vi "Load Plugin Management Core.vi"(11 "CIFPluginManager in":refnum<class "CIFPluginManager.lvclass">) -> (0 "error out":errorcluster)   [LabVIEW 2021, in "CIFPluginManager.lvclass"]
uses:
  CIFPluginManager.lvclass
  CIFPluginManager.lvclass/CIFPluginManager.ctl
  gRPC/CIF_Manager_server/RPC Service/Manager/Manager.lvclass
  C:/Program Files/National Instruments/LabVIEW 2021/vi.lib/gRPC/LabVIEW gRPC Servicer/ServiceBase/ServiceBase.lvclass
  gRPC/CIF_Manager_server/RPC Service/Manager/Manager.lvclass/Manager.ctl
  gRPC/CIF_Manager_server/RPC Messages/cif_manager_LoadPluginResponse.ctl
  gRPC/CIF_Manager_server/RPC Messages/cif_common_Status.ctl
  typedef/Plugin Load Command.ctl
  typedef/Loader Type.ctl
  <vilib>/Utility/miscctls.llb/LVMapReplaceAction.ctl
  <vilib>/CIF Foundation/CIF Core/CIFCore/Common/Typedef/Errors.ctl
  typedef/Loader Load Command.ctl
  gRPC/CIF_Manager_server/RPC Messages/cif_manager_AbortPluginResponse.ctl
  gRPC/CIF_Manager_server/RPC Messages/cif_manager_AbortAllPluginsResponse.ctl
  gRPC/CIF_Manager_server/RPC Messages/Get cif_manager_LoadPluginRequest.vi
  gRPC/CIF_Manager_server/RPC Messages/Set cif_manager_LoadPluginResponse.vi
  <vilib>/CIF Foundation/CIF Utilities/Errors/Append Error Location.vi
  gRPC/CIF_Manager_server/RPC Messages/Get cif_manager_AbortPluginRequest.vi
  gRPC/CIF_Manager_server/RPC Messages/Set cif_manager_AbortPluginResponse.vi
  gRPC/CIF_Manager_server/RPC Messages/Get cif_manager_AbortAllPluginsRequest.vi
  gRPC/CIF_Manager_server/RPC Messages/Set cif_manager_AbortAllPluginsResponse.vi
  gRPC/CIF_Manager_server/RPC Messages/Get cif_manager_LoadPluginRequest.vi/2ed25e12-861d-4677-8ead-ace2906b2041.vi
  gRPC/CIF_Manager_server/RPC Messages/FlatToRichcif_manager_LoadPluginRequest.vi
  gRPC/CIF_Manager_server/RPC Messages/Set cif_manager_LoadPluginResponse.vi/dcc74a39-081a-4bdd-860b-8ed792803c96.vi
  gRPC/CIF_Manager_server/RPC Messages/RichToFlatcif_manager_LoadPluginResponse.vi
  gRPC/CIF_Manager_server/RPC Messages/Get cif_manager_AbortPluginRequest.vi/2ed25e12-861d-4677-8ead-ace2906b2041.vi
  gRPC/CIF_Manager_server/RPC Messages/FlatToRichcif_manager_AbortPluginRequest.vi
  gRPC/CIF_Manager_server/RPC Messages/Set cif_manager_AbortPluginResponse.vi/dcc74a39-081a-4bdd-860b-8ed792803c96.vi
  gRPC/CIF_Manager_server/RPC Messages/RichToFlatcif_manager_AbortPluginResponse.vi
  gRPC/CIF_Manager_server/RPC Messages/Get cif_manager_AbortAllPluginsRequest.vi/2ed25e12-861d-4677-8ead-ace2906b2041.vi
  gRPC/CIF_Manager_server/RPC Messages/FlatToRichcif_manager_AbortAllPluginsRequest.vi
  gRPC/CIF_Manager_server/RPC Messages/Set cif_manager_AbortAllPluginsResponse.vi/dcc74a39-081a-4bdd-860b-8ed792803c96.vi
  gRPC/CIF_Manager_server/RPC Messages/RichToFlatcif_manager_AbortAllPluginsResponse.vi
  <vilib>/gRPC/LabVIEW gRPC Library/Shared/TranslateGrpcError.vi
  gRPC/CIF_Manager_server/RPC Messages/RichToFlatcif_common_Status.vi
  <vilib>/gRPC/LabVIEW gRPC Library/Server API/Server/Get Server DLL Path.vi
  <vilib>/Utility/error.llb/Error Cluster From Error Code.vi
  <vilib>/string/Create NI GUID.vi
  <vilib>/gRPC/LabVIEW gRPC Library/Server API/Message Requests/Complete Call.vi
  <vilib>/CIF Foundation/CIF Core/CIFUtilities/CIFLogs/CIFLogs.lvlib
  <vilib>/CIF Foundation/CIF Core/CIFCore/Common/CIFCoreCommon.lvlib
  <vilib>/CIF Foundation/CIF Core/CIFCore/Grpc/CIFCoreWrapper/CIFCoreWrapper.lvlib
  <vilib>/CIF Foundation/CIF Utilities/Time/Time_CIF_U.lvlib
  <vilib>/CIF Foundation/CIF Core/CIFPluginManager/gRPC/CIF_Manager_Client_Wrapper/CIFManagerClientWrapper.lvlib
  CIFPluginLoader/gRPC/CIF_Plugin_Loader_Client_Wrapper/CIFPluginLoaderClientWrapper.lvlib
  gRPC/CIF_Manager_server/CIF_Manager_server.lvlib
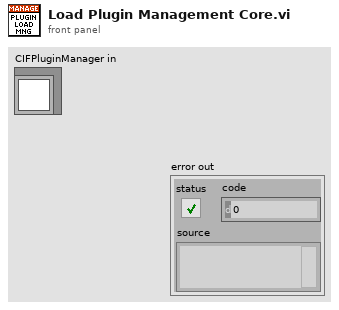
[diagram p1: front panel]
types:
  T1 = typedef "CIF_Manager_server.lvlib/Manager.lvclass/Server gRPC UEs.ctl" = cluster{"Manager LoadPlugin gRPC UE":refnum<user-event>, "Manager RegisterPlugin gRPC UE":refnum<user-event>, "Manager UnregisterPlugin gRPC UE":refnum<user-event>, "Manager QueryPluginTypes gRPC UE":refnum<user-event>, "Manager AbortPlugin gRPC UE":refnum<user-event>, "Manager UnloadAllPlugins gRPC UE":refnum<user-event>, "Manager Destroy gRPC UE":refnum<user-event>, "Manager Ping gRPC UE":refnum<user-event>, "Manager QueryErrors gRPC UE":refnum<user-event>, "Manager QueryConfig gRPC UE":refnum<user-event>, "Manager QueryInfo gRPC UE":refnum<user-event>, "Manager ResetErrorIndex gRPC UE":refnum<user-event>, "Manager ResetConfigIndex gRPC UE":refnum<user-event>, "Manager ResetInfoIndex gRPC UE":refnum<user-event>, "Manager QueryPluginInfo gRPC UE":refnum<user-event>, "Manager QueryPlugin gRPC UE":refnum<user-event>, "Manager QuerySystemStatus gRPC UE":refnum<user-event>, "Manager UpdateClock gRPC UE":refnum<user-event>, "Manager CreateOrch gRPC UE":refnum<user-event>, "Manager QueryClockStatus gRPC UE":refnum<user-event>, "Manager QueryAllChannels gRPC UE":refnum<user-event>, "Manager RegisterPluginLoader gRPC UE":refnum<user-event>, "Manager UnregisterPluginLoader gRPC UE":refnum<user-event>, "Manager CreatePluginLoader gRPC UE":refnum<user-event>, "Manager DestroyPluginLoader gRPC UE":refnum<user-event>, "Manager QueryPluginLoaders gRPC UE":refnum<user-event>}
  T2 = typedef "CIF_Manager_server.lvlib/cif_manager_LoadPluginResponse.ctl" = cluster{"status":T3}
  T3 = typedef "CIF_Manager_server.lvlib/cif_common_Status.ctl" = cluster{"code":i32, "message":string}
  T4 = typedef "CIFPluginManager.lvclass/Plugin Load Command.ctl" = cluster{"Plugin Name":string, "Plugin Path":string, "Loader Name":string, "Loader Type":T5}
  T5 = typedef "CIFPluginManager.lvclass/Loader Type.ctl" = enum16{"LabVIEW"}
  T6 = typedef "LVMapReplaceAction.ctl" = enum32{"Modify Entry only if found", "Add or Modify Entry", "Delete Entry"}
  T7 = typedef "CIFCoreCommon.lvlib/Errors.ctl" = enum16{"Invalid Clock ID", "Long Sleep", "gRPC Server Not Found", "Config Parse", "Timestamp Wrap", "Delayed Execution", "Duplicate Channel", "Missing Channel", "Incorrect Type", "Flatten Error", "Unflatten Data", "Unique Name", "Plugin Not Found", "Plugin Type Not Found", "Plugin Version Not Found", "Manager Not Found", "Numerical Issue", "Time Jump", "Clock ID Match", "Channel Length", "Plugin Connection", "gRPC Server Connection", "PPL Name Match", "Build", "Config Log Parse", "Plugin Load", "UI Subpanel Load", "Python Name", "Invalid Name", "Unable to Change Ch Buffer", "Failed Kill", "Failed SysExec", "Function Not Implemented", "Load Timeout"}
  T8 = typedef "CIFPluginManager.lvclass/Loader Load Command.ctl" = cluster{"Loader Type":T5, "Loader Name":string}
  T9 = typedef "CIF_Manager_server.lvlib/cif_manager_AbortPluginResponse.ctl" = cluster{"status":T3}
  T10 = typedef "CIF_Manager_server.lvlib/cif_manager_AbortAllPluginsResponse.ctl" = cluster{"status":T3}
  T11 = typedef "grpc-lvsupport-release.lvlib/grpcId.ctl" = u64
  T12 = typedef "CIF_Manager_server.lvlib/cif_manager_LoadPluginRequest.ctl" = cluster{"plugin_type":string, "plugin_name":string, "version":string, "loader_process":string}
  T13 = typedef "CIFPluginManager.lvclass/Discovered Plugin.ctl" = cluster{"Filename":string, "Plugin Type":string, "Qualified name":string, "Version":T14, "Plugin Metadata":T15, "Loader Type":T5, "File Path":string, "Relative Path":string[]}
  T14 = typedef "CIFCoreCommon.lvlib/Version.ctl" = cluster{"Major":i32, "Minor":i32, "Fix":i32, "Build":i32}
  T15 = typedef "CIFPluginManager.lvclass/Plugin Metadata.ctl" = cluster{"Description":string, "History":string, "Author":string}
  T16 = typedef "CIF_Manager_client.lvlib/cif_common_Status.ctl" = cluster{"code":i32, "message":string}
  T17 = typedef "CIFPluginManager.lvclass/Loader Map.ctl" = map{string, T18}
  T18 = typedef "CIFPluginManager.lvclass/Loaders.ctl" = cluster{"Loader Type":T5, "grpc_port":i32, "pid":u32, "gRPC ID":T11, "Load Timestamp":i64, "Unloading":bool, "Ready for removal":bool, "Unload Timestamp":i64}
  T19 = typedef "CIFPluginManager.lvclass/Plugin Management Data Map.ctl" = map{string, T20}
  T20 = typedef "CIFPluginManager.lvclass/Plugin Management Data.ctl" = cluster{"Unique Name":string, "Plugin Type":string, "gRPC Port":i32, "gRPC ID":T11, "Loader Type":T5, "Loader":string, "Version":T14, "Load Timestamp":i64, "Unload Timestamp":i64, "Unloading":bool, "Ready for removal":bool, "status":T21, "channels":T30}
  T21 = typedef "CIF_Manager_server.lvlib/cif_management_common_PluginStatusData.ctl" = cluster{"state":T22, "timing_statistics":T23, "fifo_statistics":T25, "error":T26, "monitor_doubles":T27, "monitor_u64s":T28, "monitor_i64s":T29}
  T22 = typedef "CIF_Manager_server.lvlib/cif_management_common_PluginStatusData_PluginState.ctl" = enum32{"PLUGINSTATE_UNKNOWN", "PLUGINSTATE_CREATING", "PLUGINSTATE_LISTENING", "PLUGINSTATE_RUNNING", "PLUGINSTATE_CLEANINGUP", "PLUGINSTATE_DESTROYING"}
  T23 = typedef "CIF_Manager_server.lvlib/cif_management_common_TimingStatistics.ctl" = cluster{"period":T24, "wake_error":T24, "execute":T24, "housekeep":T24, "idle":T24, "cleanup":T24, "custom_1":T24, "custom_2":T24}
  T24 = typedef "CIF_Manager_server.lvlib/cif_common_TimingStats.ctl" = cluster{"max":i64, "min":i64, "avg":dbl}
  T25 = typedef "CIF_Manager_server.lvlib/cif_management_common_FifoStatistics.ctl" = cluster{"from_t0":T24, "from_previous_plugin":T24, "output_error":T24}
  T26 = typedef "CIF_Manager_server.lvlib/cif_management_common_Error.ctl" = cluster{"status":bool, "code":i32}
  T27 = typedef "CIF_Manager_server.lvlib/cif_management_common_MonitorDoubles.ctl" = cluster{"double_1":dbl, "double_2":dbl, "double_3":dbl, "double_4":dbl}
  T28 = typedef "CIF_Manager_server.lvlib/cif_management_common_MonitorU64.ctl" = cluster{"u64_1":u64, "u64_2":u64, "u64_3":u64, "u64_4":u64}
  T29 = typedef "CIF_Manager_server.lvlib/cif_management_common_MonitorI64.ctl" = cluster{"i64_1":i64, "i64_2":i64, "i64_3":i64, "i64_4":i64}
  T30 = typedef "CIF_Manager_server.lvlib/cif_management_common_Channels.ctl" = cluster{"channels":T31[]}
  T31 = typedef "CIF_Manager_server.lvlib/cif_management_common_Channel.ctl" = cluster{"name":string, "direction":T32, "type":string, "custom_config":u8[], "connected":bool, "connected_name":string, "forced":bool, "channel_pattern":T33}
  T32 = typedef "CIF_Manager_server.lvlib/cif_management_common_ChannelDirection.ctl" = enum32{"CHANNELDIRECTION_UNKNOWN", "CHANNELDIRECTION_PUBLISHER", "CHANNELDIRECTION_SUBSCRIBER"}
  T33 = typedef "CIF_Manager_server.lvlib/cif_management_common_ChannelPattern.ctl" = enum32{"CHANNELPATTERN_UNKNOWN", "CHANNELPATTERN_TAG", "CHANNELPATTERN_FIFO", "CHANNELPATTERN_MULTIFIFO", "CHANNELPATTERN_BACKPRESSUREFIFO"}
  T34 = typedef "CIF_Manager_server.lvlib/cif_manager_AbortPluginRequest.ctl" = cluster{"plugin_name":string}
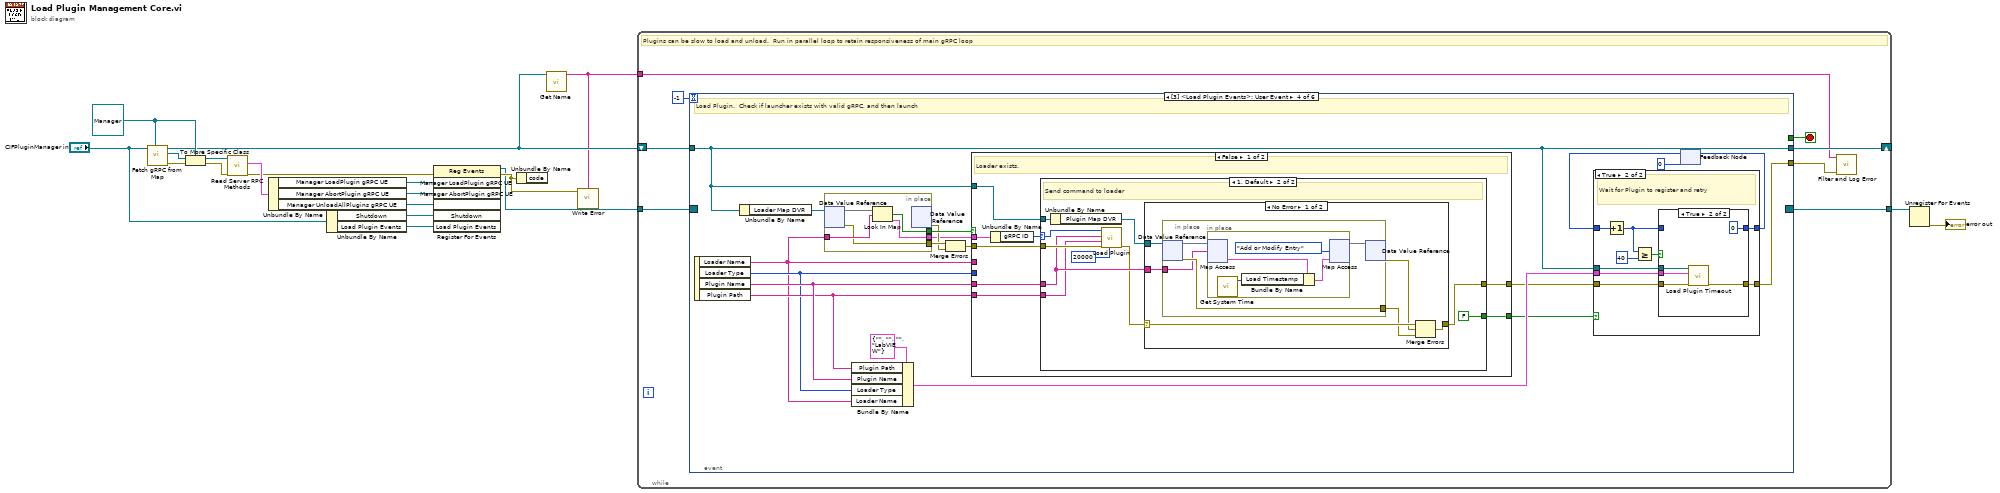
[diagram p0: block diagram]
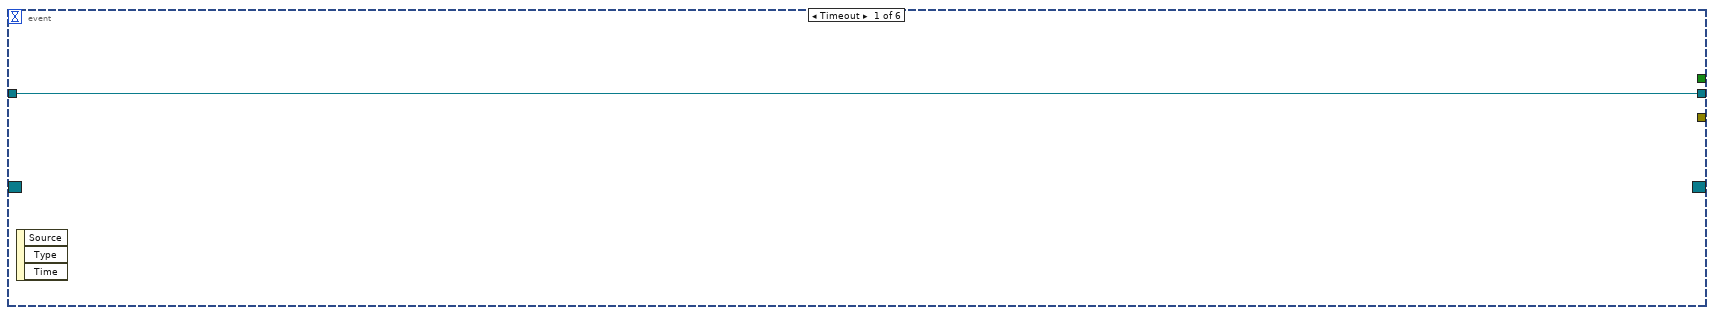
[diagram p2: hidden frame]
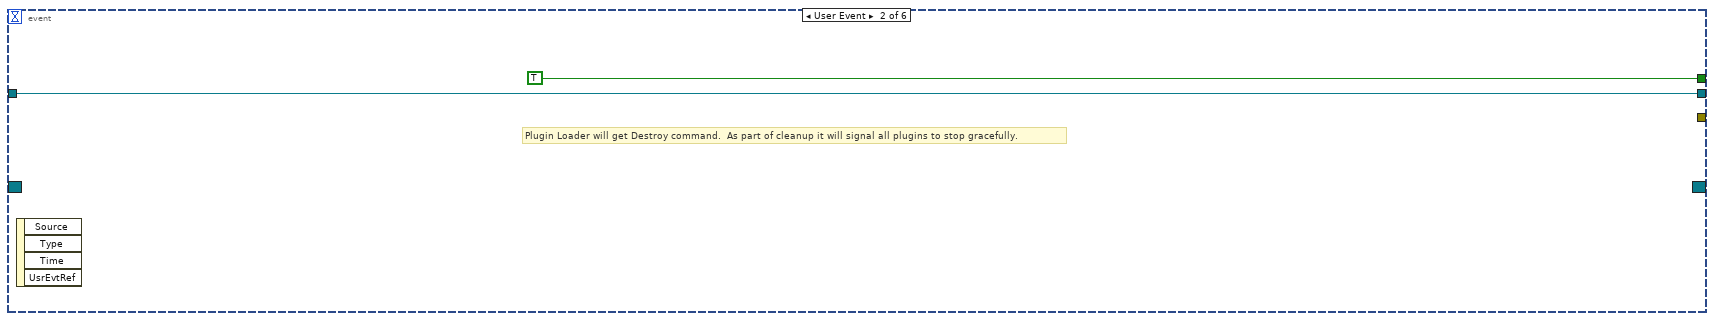
[diagram p3: hidden frame]
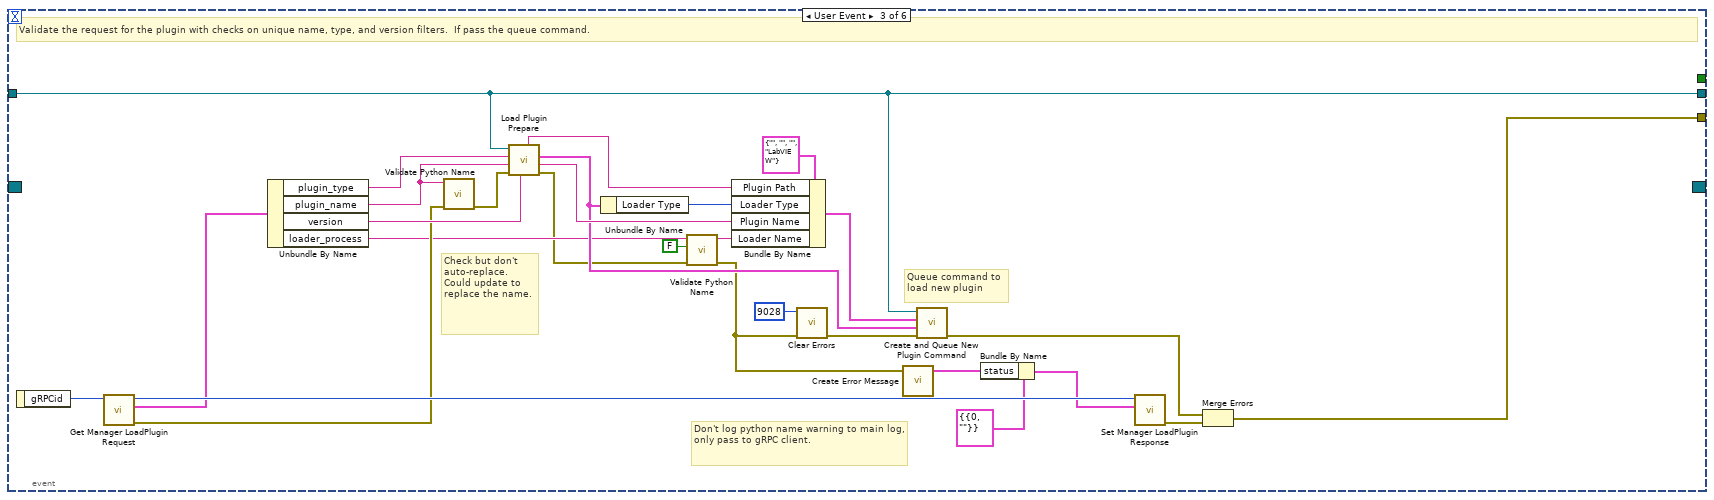
[diagram p4: hidden frame]
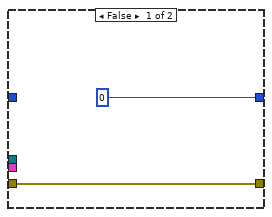
[diagram p5: hidden frame]
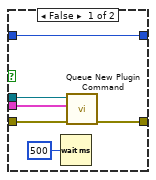
[diagram p6: hidden frame]
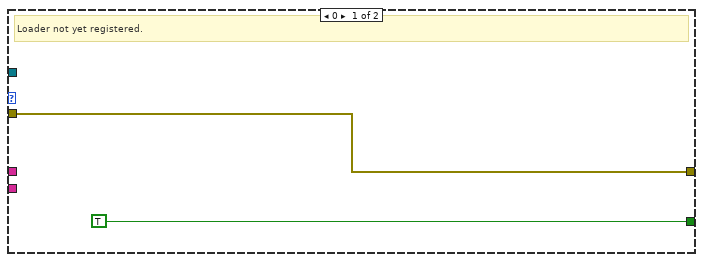
[diagram p7: hidden frame]
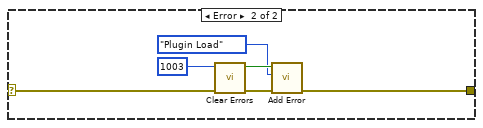
[diagram p8: hidden frame]
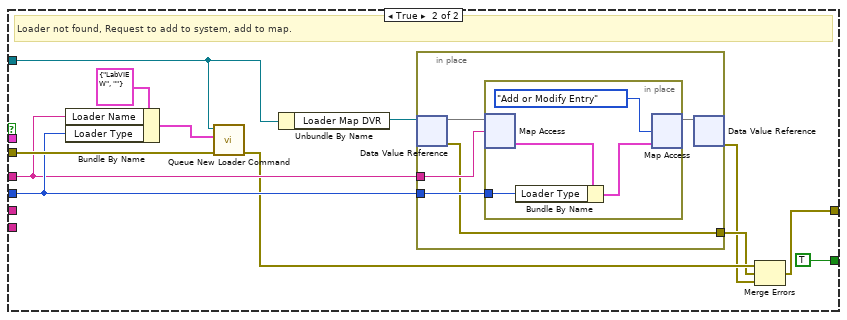
[diagram p9: hidden frame]
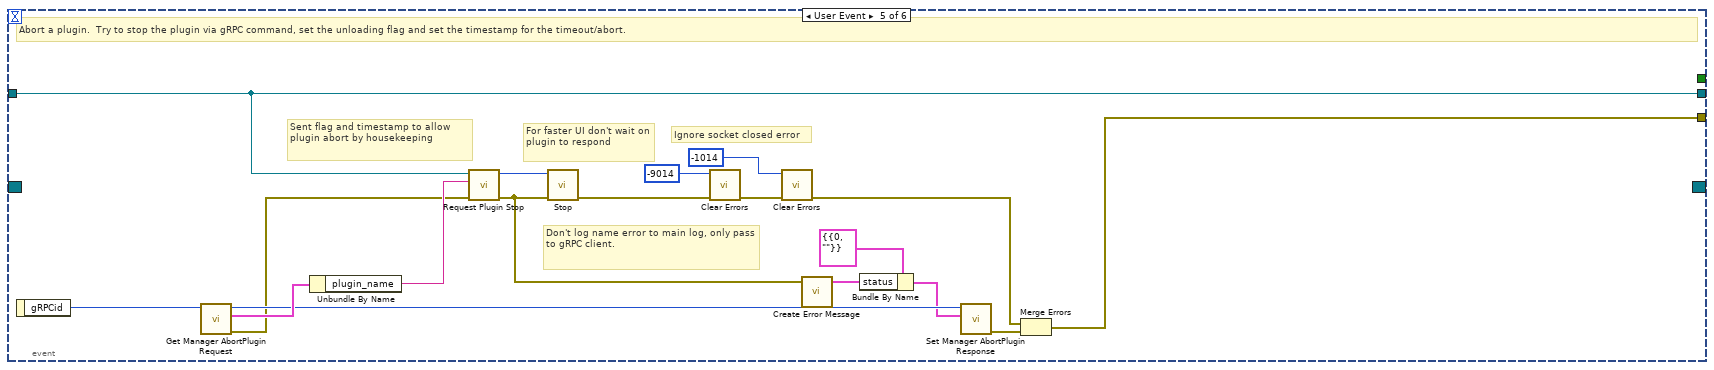
[diagram p10: hidden frame]
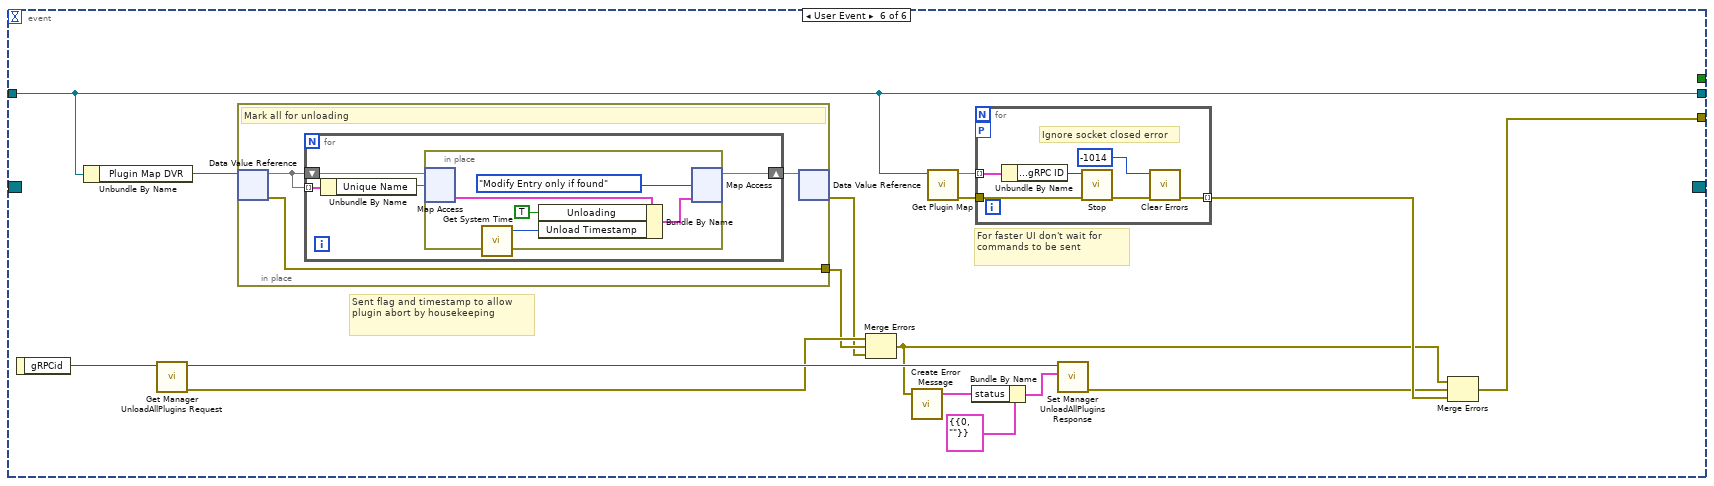
[diagram p11: hidden frame]
diagram:
  w16 = refnum<class "Manager.lvclass"> refnum ("CIF_Manager_server.lvlib:Manager.lvclass")
  n1 = call "Fetch gRPC from Map.vi"("gRPC Server Class type"=w16, "Plugin Manager in"="CIFPluginManager in") -> ("error out"=w15:errorcluster, "gRPC Server Class out"=w17:refnum<class "ServiceBase.lvclass">, "Plugin Manager out"=w2:refnum<class "CIFPluginManager.lvclass">)  [unwired: 7 in]
  n2 = To More Specific Class(target class=w16, reference=w17, error in=w15) -> (specific class reference=w13:refnum<class "Manager.lvclass">, error out=w14:errorcluster)
  n3 = call "Read Server RPC Methods.vi"("error in (no error)"=w14, "gRPC service in"=w13) -> ("error out"=w8:errorcluster, "Server RPC Methods"=w9:T1)  [unwired: 7 in, 1 out]
  n4 = Unbundle By Name(w9) -> ("Manager LoadPlugin gRPC UE"=w4:refnum<user-event>, "Manager AbortPlugin gRPC UE"=w5:refnum<user-event>, "Manager UnloadAllPlugins gRPC UE"=w6:refnum<user-event>)
  n5 = Unbundle By Name("CIFPluginManager in") -> ("Shutdown"=w7:refnum<user-event>, "Load Plugin Events"=w3:refnum<user-event>)
  n6 = register-events(error in=w8, w4, w5, w6, w7, w3) -> (reference out=w10:refnum<event-registration>, error out=w11:errorcluster)  [unwired: 1 in]
  n7 = Unbundle By Name(w11) -> ()  [unwired: 1 out]
  n8 = call "Get Name.vi"("CIFPluginManager in"=w2) -> ("Name"=w1:string)  [unwired: 10 in]
  n9 = call <vilib>:"Write Error.vi"("error in (no error)"=w11, "Plugin Name"=w1) -> ()  [unwired: 2 in, 1 out]
  n10 = while {
    tunnel: w10 -> [w21]
    shift-right: [w23] -> _
    shift-left: w2 -> [w27]
    tunnel: [w24] -> w18
    tunnel: w1 -> [w20]
    stop <- w25 stop-if-true
    # "Plugins can be slow to load and unload.  Run in parallel loop to retain responsiveness of main gRPC loop"
    n11 = event shown="[3] <Load Plugin Events>: User Event" {
      selector: w21 -> [_ _ _ _ _ _]
      dyn-events: [_ _ _ _ _ _] -> w24
      timeout: -1 -> [_ _ _ _ _ _]
      tunnel: w27 -> [w28 w29 w42 w63 w176 w193]
      tunnel: [w28 w29 w42 w63 w176 w193] -> w23
      tunnel: [_ TRUE _ _ _ _] -> w25
      tunnel: [_ _ w51 w59 w178 w190] -> w22
      event Timeout {
        n12 = event-data() -> ()  [unwired: 1 in, 3 out]
      }
      event User Event {
        # "Plugin Loader will get Destroy command.  As part of cleanup it will signal all plugins to stop gracefully."
        n13 = event-data() -> ()  [unwired: 1 in, 4 out]
      }
      event User Event {
        # "Queue command to load new plugin"
        # "Don't log python name warning to main log, only pass to gRPC client."
        # "Check but don't auto-replace.  Could update to replace the name."
        # "Validate the request for the plugin with checks on unique name, type, and version filters.  If pass the queue command."
        n14 = event-data() -> ("gRPCid"=w50:T11)  [unwired: 1 in]
        n15 = call "Get Manager LoadPlugin Request.vi"("gRPCid"=w50) -> ("error out"=w52:errorcluster, "Message Data"=w56:T12, "gRPCid out"=w58:T11)  [unwired: 8 in]
        n16 = Unbundle By Name(w56) -> ("plugin_type"=w39:string, "plugin_name"=w53:string, "version"=w55:string, "loader_process"=w38:string)
        n17 = call <vilib>:"Validate Python Name.vi"("error in (no error)"=w52, "Name In"=w53) -> ("error out"=w54:errorcluster)  [unwired: 8 in, 1 out]
        n18 = call "Load Plugin Prepare.vi"("Version String"=w55, "error in (no error)"=w54, "Unique Name"=w53, "Plugin Type"=w39, "CIFPluginManager in"=w42) -> ("error out"=w35:errorcluster, "Unique Name (dup)"=w43:string, "Matching Plugin"=w41:T13, "path"=w45:string)  [unwired: 3 in]
        n19 = Unbundle By Name(w41) -> ("Loader Type"=w44:T5)
        n20 = call <vilib>:"Validate Python Name.vi"("error in (no error)"=w35, "GUID for Empty"=FALSE, "Name In"=w38) -> ("error out"=w34:errorcluster, "Valid Name"=w37:string)  [unwired: 7 in]
        n21 = Bundle By Name(cluster=T4 {"Plugin Name"="", "Plugin Path"="", "Loader Name"="", "Loader Type"=enum."LabVIEW"} ("New Plugin"), "Plugin Path"=w45, "Loader Type"=w44, "Plugin Name"=w43, "Loader Name"=w37) -> (w47:T4)
        n22 = call <vilib>:"Clear Errors.vi"("error in (no error)"=w34, "specific error code to clear (0: all)"=9028) -> ("error out"=w48:errorcluster)  [unwired: 4 in, 1 out]
        n23 = call "Create Error Message.vi"("error in (no error)"=w34) -> ("Error Message"=w32:T16)  [unwired: 3 in]
        n24 = call "Create and Queue New Plugin Command.vi"("error in (no error)"=w48, "Matching Plugin"=w41, "New Plugin"=w47, "CIFPluginManager in"=w42) -> ("error out"=w40:errorcluster)  [unwired: 7 in]
        n25 = Bundle By Name(cluster=T2 {"status"={"code"=0, "message"=""}} ("Message Data"), "status"=w32) -> (w31:T2)
        n26 = call "Set Manager LoadPlugin Response.vi"("Message Data"=w31, "gRPCid in"=w58) -> ("error out"=w57:errorcluster)  [unwired: 9 in]
        n27 = Merge Errors(w40, w57) -> (w51:errorcluster)
      }
      event User Event {
        # "Load Plugin.  Check if launcher exists with valid gRPC, and then launch"
        n28 = event-data() -> ("Loader Name"=w67:string, "Loader Type"=w68:T5, "Plugin Name"=w70:string, "Plugin Path"=w69:string)  [unwired: 1 in]
        n29 = Unbundle By Name(w63) -> ("Loader Map DVR"=w77:refnum<data-value>)
        n30 = in-place {
          in-place-border: w67 -> [w164]
          in-place-border: [w163] -> w75
          in-place-border: [w162] -> w72
          in-place-border: [w161] -> w76
          n31 = in-place-dvr #1(w77) -> (w165:T17, w163:errorcluster)
          n32 = Look In Map(map=w165, key=w164) -> (key not found?=w161:bool, value=w162:T18)  [unwired: 1 in]
          n33 = in-place-dvr #1() -> (w74:errorcluster)  [unwired: 1 in, 1 out]
        }
        n34 = Bundle By Name(cluster=T4 {"Plugin Name"="", "Plugin Path"="", "Loader Name"="", "Loader Type"=enum."LabVIEW"} ("New Plugin"), "Plugin Path"=w69, "Plugin Name"=w70, "Loader Type"=w68, "Loader Name"=w67) -> (w62:T4)
        n35 = Merge Errors(w75, w74) -> (w73:errorcluster)
        n36 = case shown="False" w76 {
          tunnel: w63 -> [w100 w147]
          tunnel: w73 -> [w101 w151]
          tunnel: [w102 w140] -> w61
          tunnel: w68 -> [_ w145]
          tunnel: w67 -> [_ w144]
          tunnel: [w105 TRUE] -> w60
          tunnel: w72 -> [w107 _]
          tunnel: w70 -> [w104 _]
          tunnel: w69 -> [w103 _]
          frame False {
            # "Loader exists."
            n37 = Unbundle By Name(w107) -> ("gRPC ID"=w106:T11)
            n38 = case shown="1, Default" w106 {
              selector: w106 -> [_ w119]
              tunnel: [TRUE FALSE] -> w105
              tunnel: w104 -> [_ w115]
              tunnel: w103 -> [_ w114]
              tunnel: [w108 w116] -> w102
              tunnel: w101 -> [w108 w118]
              tunnel: w100 -> [_ w113]
              frame 0 {
                # "Loader not yet registered."
              }
              frame 1, Default {
                # "Send command to loader"
                n39 = Unbundle By Name(w113) -> ("Plugin Map DVR"=w111:refnum<data-value>)
                n40 = call "Load Plugin.vi"("timeout (ms)"=20000, "error in"=w118, "Plugin Path"=w114, "Plugin Name"=w115, "gRPC ID in"=w119) -> ("error out"=w112:errorcluster)  [unwired: 5 in, 1 out]
                n41 = case shown="No Error" w112 {
                  selector: w112 -> [w124 w135]
                  tunnel: w115 -> [w125 _]
                  tunnel: [w121 w134] -> w116
                  tunnel: w111 -> [w120 _]
                  frame No Error {
                    n42 = in-place {
                      in-place-border: w125 -> [w127]
                      in-place-border: [w129] -> w123
                      n43 = in-place-dvr #2(w120) -> (w128:T19, w129:errorcluster)
                      n44 = in-place {
                        n45 = in-place-map #3(w128, w127) -> (w133:T20)  [unwired: 1 in, 1 out]
                        n46 = call <vilib>:"Get System Time.vi"() -> ("Time (ns)"=w130:i64)  [unwired: 5 in]
                        n47 = Bundle By Name(cluster=w133, "Load Timestamp"=w130) -> (w132:T20)
                        n48 = in-place-map #3(w132, LVMapReplaceAction."Add or Modify Entry" ("action")) -> (w126:T19)  [unwired: 2 out]
                      }
                      n49 = in-place-dvr #2(w126) -> (w122:errorcluster)  [unwired: 1 out]
                    }
                    n50 = Merge Errors(w124, w122, w123) -> (w121:errorcluster)
                  }
                  frame Error {
                    n51 = call <vilib>:"Clear Errors.vi"("error in (no error)"=w135, "specific error code to clear (0: all)"=1003) -> ("error out"=w139:errorcluster, "specific error cleared?"=w138:bool)  [unwired: 4 in]
                    n52 = call <vilib>:"Add Error.vi"("error in (no error)"=w139, "Error"=Errors."Plugin Load", "Insert Error"=w138) -> ("error out"=w134:errorcluster)  [unwired: 8 in]
                  }
                }
              }
            }
          }
          frame True {
            # "Loader not found, Request to add to system, add to map."
            n53 = Bundle By Name(cluster=T8 {"Loader Type"=enum."LabVIEW", "Loader Name"=""} ("New Launcher"), "Loader Name"=w144, "Loader Type"=w145) -> (w149:T8)
            n54 = call "Queue New Loader Command.vi"("error in (no error)"=w151, "New Launcher"=w149, "CIFPluginManager in"=w147) -> ("error out"=w143:errorcluster)  [unwired: 8 in]
            n55 = Unbundle By Name(w147) -> ("Loader Map DVR"=w146:refnum<data-value>)
            n56 = in-place {
              in-place-border: w145 -> [w154]
              in-place-border: w144 -> [w153]
              in-place-border: [w152] -> w142
              n57 = in-place-dvr #4(w146) -> (w156:T17, w152:errorcluster)
              n58 = in-place {
                in-place-border: w154 -> [w157]
                n59 = in-place-map #5(w156, w153) -> (w159:T18)  [unwired: 1 in, 1 out]
                n60 = Bundle By Name(cluster=w159, "Loader Type"=w157) -> (w158:T18)
                n61 = in-place-map #5(w158, LVMapReplaceAction."Add or Modify Entry" ("action")) -> (w155:T17)  [unwired: 2 out]
              }
              n62 = in-place-dvr #4(w155) -> (w141:errorcluster)  [unwired: 1 out]
            }
            n63 = Merge Errors(w143, w142, w141) -> (w140:errorcluster)
          }
        }
        n64 = feedback #6(0) -> (w66:i32)
        n65 = case shown="True" w60 {
          tunnel: w61 -> [w79 w86]
          tunnel: w63 -> [_ w88]
          tunnel: w62 -> [_ w87]
          tunnel: [w79 w85] -> w59
          tunnel: w66 -> [_ w84]
          tunnel: [0 w80] -> w64
          frame False {
          }
          frame True {
            # "Wait for Plugin to register and retry"
            n66 = Increment(x=w84) -> (x+1=w81:i32)
            n67 = Greater Or Equal?(x=w81, y=40) -> (x >= y?=w83:bool)
            n68 = case shown="True" w83 {
              tunnel: w88 -> [w91 w95]
              tunnel: w87 -> [w90 w96]
              tunnel: w86 -> [w93 w98]
              tunnel: [w92 w97] -> w85
              tunnel: w81 -> [w89 _]
              tunnel: [w89 0] -> w80
              frame False {
                n69 = Wait (ms)(milliseconds to wait=u32 500) -> ()  [unwired: 1 out]
                n70 = call "Queue New Plugin Command.vi"("error in (no error)"=w93, "New Plugin"=w90, "CIFPluginManager in"=w91) -> ("error out"=w92:errorcluster)  [unwired: 8 in]
              }
              frame True {
                n71 = call "Load Plugin Timeout.vi"("error in (no error)"=w98, "New Plugin"=w96, "CIFPluginManager in"=w95) -> ("error out"=w97:errorcluster)  [unwired: 8 in]
              }
            }
          }
        }
        n72 = feedback-in #6(w64) -> ()
      }
      event User Event {
        # "Sent flag and timestamp to allow plugin abort by housekeeping"
        # "Ignore socket closed error"
        # "Don't log name error to main log, only pass to gRPC client."
        # "For faster UI don't wait on plugin to respond"
        # "Abort a plugin.  Try to stop the plugin via gRPC command, set the unloading flag and set the timestamp for the timeout/abort."
        n73 = event-data() -> ("gRPCid"=w179:T11)  [unwired: 1 in]
        n74 = call "Get Manager AbortPlugin Request.vi"("gRPCid"=w179) -> ("error out"=w177:errorcluster, "Message Data"=w182:T34, "gRPCid out"=w180:T11)  [unwired: 8 in]
        n75 = Unbundle By Name(w182) -> ("plugin_name"=w183:string)
        n76 = call "Request Plugin Stop.vi"("error in (no error)"=w177, "Unique Name"=w183, "CIFPluginManager in"=w176) -> ("error out"=w174:errorcluster, "gRPC ID"=w175:T11)  [unwired: 7 in]
        n77 = call <vilib>:"Stop.vi"("error in"=w174, "gRPC ID"=w175) -> ("error out"=w172:errorcluster)  [unwired: 8 in, 1 out]
        n78 = call <vilib>:"Clear Errors.vi"("error in (no error)"=w172, "specific error code to clear (0: all)"=-9014) -> ("error out"=w170:errorcluster)  [unwired: 4 in, 1 out]
        n79 = call <vilib>:"Clear Errors.vi"("error in (no error)"=w170, "specific error code to clear (0: all)"=-1014) -> ("error out"=w169:errorcluster)  [unwired: 4 in, 1 out]
        n80 = call "Create Error Message.vi"("error in (no error)"=w174) -> ("Error Message"=w167:T16)  [unwired: 3 in]
        n81 = Bundle By Name(cluster=T9 {"status"={"code"=0, "message"=""}} ("Message Data"), "status"=w167) -> (w166:T9)
        n82 = call "Set Manager AbortPlugin Response.vi"("Message Data"=w166, "gRPCid in"=w180) -> ("error out"=w181:errorcluster)  [unwired: 9 in]
        n83 = Merge Errors(w169, w181) -> (w178:errorcluster)
      }
      event User Event {
        # "Sent flag and timestamp to allow plugin abort by housekeeping"
        # "For faster UI don't wait for commands to be sent"
        n84 = event-data() -> ("gRPCid"=w198:T11)  [unwired: 1 in]
        n85 = Unbundle By Name(w193) -> ("Plugin Map DVR"=w199:refnum<data-value>)
        n86 = call "Get Manager UnloadAllPlugins Request.vi"("gRPCid"=w198) -> ("error out"=w196:errorcluster, "gRPCid out"=w197:T11)  [unwired: 8 in, 1 out]
        n87 = in-place {
          in-place-border: [w206] -> w195
          # "Mark all for unloading"
          n88 = in-place-dvr #7(w199) -> (w208:T19, w206:errorcluster)
          n89 = for {
            tunnel: w208 -> [w210] mode=indexing
            shift-right: [w211] -> w207
            shift-left: w208 -> [w212]
            n90 = Unbundle By Name(w210) -> ("Unique Name"=w209:string)
            n91 = in-place {
              n92 = in-place-map #8(w212, w209) -> (w214:T20)  [unwired: 1 in, 1 out]
              n93 = call <vilib>:"Get System Time.vi"() -> ("Time (ns)"=w215:i64)  [unwired: 5 in]
              n94 = Bundle By Name(cluster=w214, "Unloading"=TRUE, "Unload Timestamp"=w215) -> (w213:T20)
              n95 = in-place-map #8(w213, LVMapReplaceAction."Modify Entry only if found" ("action")) -> (w211:T19)  [unwired: 2 out]
            }
          }
          n96 = in-place-dvr #7(w207) -> (w194:errorcluster)  [unwired: 1 out]
        }
        n97 = Merge Errors(w196, w195, w194) -> (w188:errorcluster)
        n98 = call "Create Error Message.vi"("error in (no error)"=w188) -> ("Error Message"=w185:T16)  [unwired: 3 in]
        n99 = call "Get Plugin Map.vi"("CIFPluginManager in"=w193) -> ("error out"=w191:errorcluster, "Plugin Map"=w192:T19)  [unwired: 9 in]
        n100 = Bundle By Name(cluster=T10 {"status"={"code"=0, "message"=""}} ("Message Data"), "status"=w185) -> (w184:T10)
        n101 = for {
          tunnel: w191 -> [w203]
          tunnel: w192 -> [w204] mode=indexing
          workers-P: _ -> [_]
          tunnel: [w201] -> w189 mode=indexing
          # "Ignore socket closed error"
          n102 = Unbundle By Name(w204) -> ("Plugin Management Data.gRPC ID"=w205:T11)
          n103 = call <vilib>:"Stop.vi"("error in"=w203, "gRPC ID"=w205) -> ("error out"=w202:errorcluster)  [unwired: 8 in, 1 out]
          n104 = call <vilib>:"Clear Errors.vi"("error in (no error)"=w202, "specific error code to clear (0: all)"=-1014) -> ("error out"=w201:errorcluster)  [unwired: 4 in, 1 out]
        }
        n105 = call "Set Manager UnloadAllPlugins Response.vi"("Message Data"=w184, "gRPCid in"=w197) -> ("error out"=w187:errorcluster)  [unwired: 9 in]
        n106 = Merge Errors(w188, w187, w189) -> (w190:errorcluster)
      }
    }
    n107 = call <vilib>:"Filter and Log Error.vi"("error In"=w22, "Name"=w20) -> ()  [unwired: 10 in]
  }
  n108 = Unregister For Events(event registration refnum=w18) -> (error out=→"error out":errorcluster)  [unwired: 1 in]
